vi "Assert Array Not Empty.vi"(4 "Execution time (s)":dbl=-1.0, 5 "Assert Only? (F)":bool, 6 "error code (1)":i32=1, 7 "Label (\"\")":string, 8 "error in (no error)":errorcluster, 9 "Register with caller test (F)":bool, 11 "Array":variant) -> (0 "error out":errorcluster, 2 "Properties.Assert":refnum<class "Properties.Assert.lvclass">)   [LabVIEW 2013, in "Caraya.lvlib" / "Assert.lvclass"]
doc: "Asserts that an array is not empty."
uses:
  Assert.lvclass
  Properties.Assert/Properties.Assert.lvclass
  Properties/Properties.lvclass
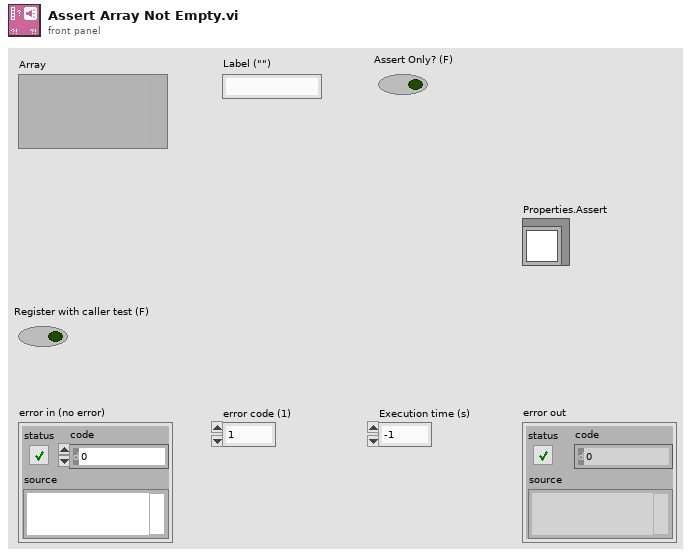
[diagram p1: front panel]
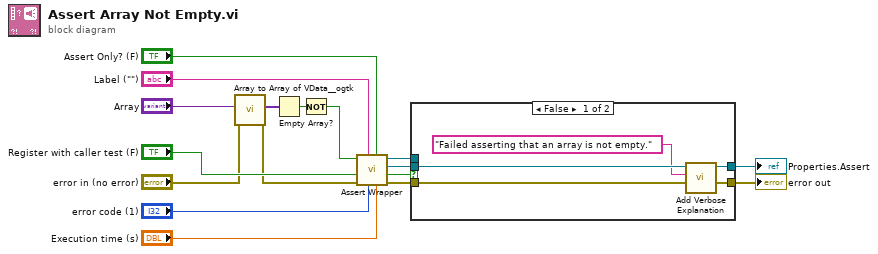
[diagram p0: block diagram]
diagram:
  n1 = call <userlib>:"Array to Array of VData__ogtk.vi"("error in (no error)"="error in (no error)", "MultiD Array"="Array") -> ("error out"=w4:errorcluster, "1D Array of Variants"=w3:variant[])  [unwired: 8 in]
  n2 = Empty Array?(array=w3) -> (empty?=w2:bool)
  n3 = Not(x=w2) -> (.not. x?=w1:bool)
  n4 = call "Assert Wrapper.vi"("Execution time (s)"="Execution time (s)", "Assert Only? (F)"="Assert Only? (F)", "error code (1)"="error code (1)", "Label"="Label (\"\")", "error in (no error)"=w4, "Register with caller test (F)"="Register with caller test (F)", "Assert?"=w1) -> ("error out"=w8:errorcluster, "Verbose"=w12:bool, "Properties.Assert"=w10:refnum<class "Properties.Assert.lvclass">, "Assert out"=w11:refnum<class "Assert.lvclass">)  [unwired: 1 in]
  n5 = case shown="False" w12 {
    tunnel: w11 -> [_ _]
    tunnel: w10 -> [w20 w24]
    tunnel: [w21 w23] -> w9
    tunnel: w8 -> [w22 w23]
    tunnel: [w19 w24] -> w7
    frame False {
      n6 = call "Add Verbose Explanation.vi"("error in (no error)"=w22, "Verbose Explanation"="Failed asserting that an array is not empty.", "Properties"=w20) -> ("error out"=w21:errorcluster, "Properties"=w19:refnum<class "Properties.Assert.lvclass">)  [unwired: 7 in]
    }
    frame True {
    }
  }
  "error out" <- w9
  "Properties.Assert" <- w7
